vi "Obtain Log Queue.vi"(8 "error in":errorcluster) -> (0 "error out":errorcluster, 3 "queue out":refnum<queue>)   [LabVIEW 2018]
uses:
  Huskie Board.ctl
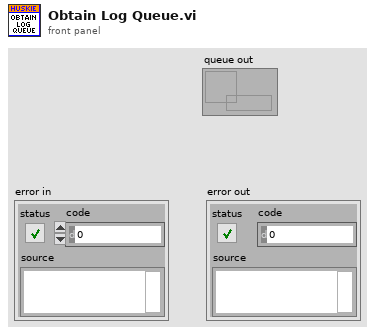
[diagram p1: front panel]
types:
  T1 = typedef "Huskie Board.ctl" = enum16{"Huskie Board", "Logging Queue"}
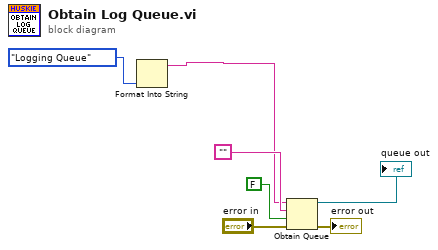
[diagram p0: block diagram]
diagram:
  n1 = Format Into String(Huskie_Board."Logging Queue") -> (resulting string=w2:string)  [unwired: 3 in, 1 out]
  n2 = Obtain Queue(name (unnamed)=w2, element data type="", create if not found? (T)=FALSE, error in (no error)="error in") -> (queue out=→"queue out":refnum<queue>, error out=→"error out":errorcluster)  [unwired: 1 in, 1 out]
